vi "half width of array cut at peak.vi"(9 "0.5 means FWHM":dbl=0.5 format="%#_13g", 10 "amplitude value biggest peak":dbl, 11 "counts":dbl[](graph)) -> (3 "half width half max":dbl)   [LabVIEW 2020]
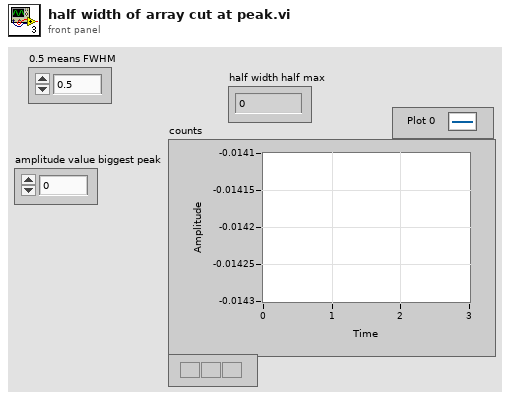
[diagram p1: front panel]
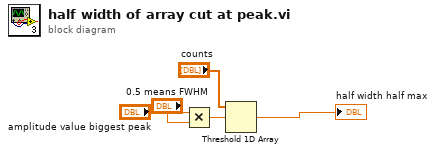
[diagram p0: block diagram]
diagram:
  n1 = Multiply(x="amplitude value biggest peak", y="0.5 means FWHM") -> (x*y=w4:dbl)
  n2 = Threshold 1D Array(2:w4, 3:"counts") -> (0:→"half width half max":dbl)  [unwired: 1 in]
